vi "MathLink.vi"(2 "Arg":variant, 3 "Action":enum16{"Open", "Answer", "Close"}(ring), 4 "mlp in":u64) -> (0 "Status":i32, 1 "mlp out":u64)   [LabVIEW 2014]
uses:
  ml64i4.dll
panel:
  in  "VIs":variant
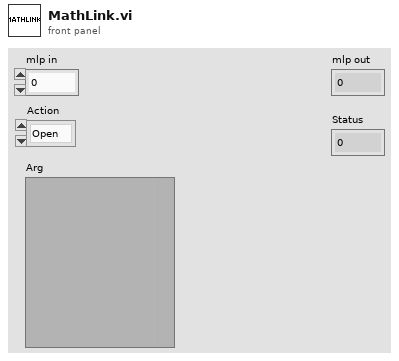
[diagram p1: front panel]
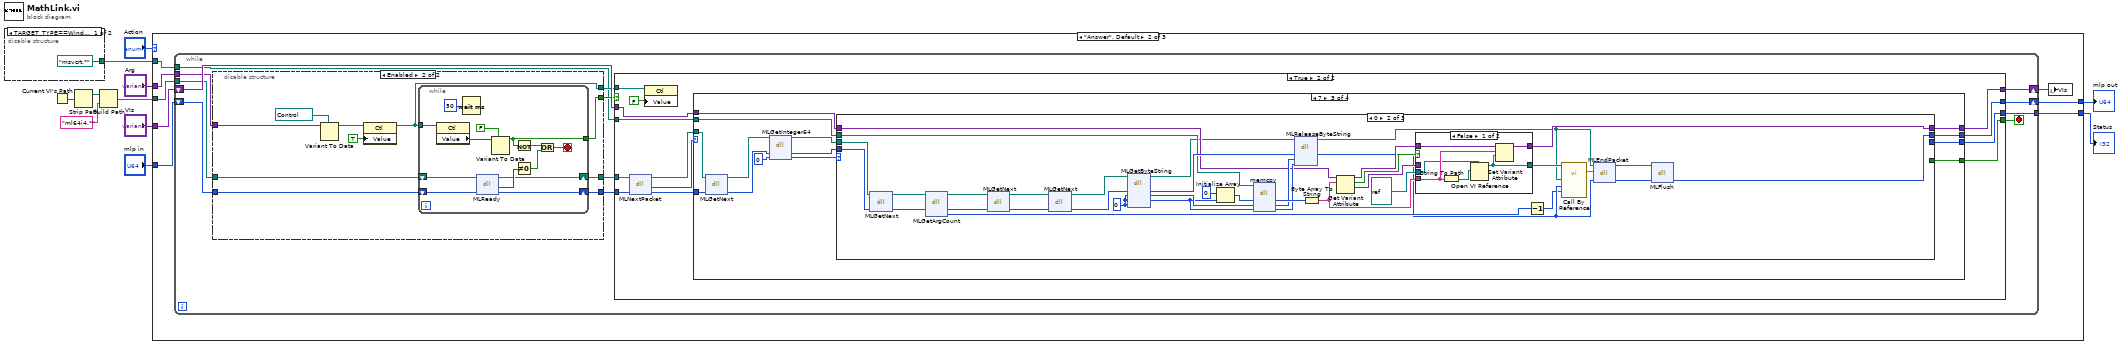
[diagram p0: block diagram]
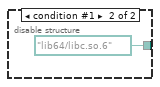
[diagram p2: hidden frame]
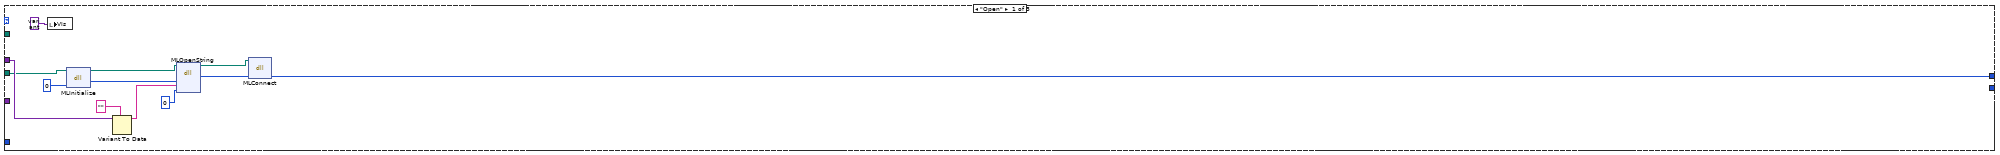
[diagram p3: hidden frame]
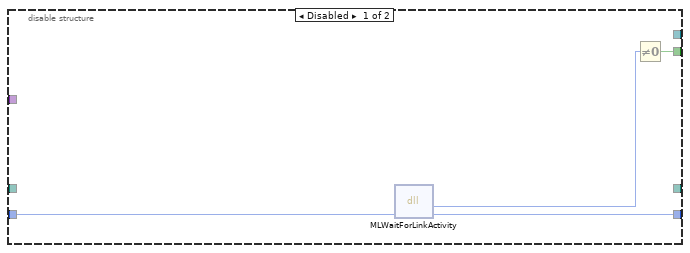
[diagram p4: hidden frame]
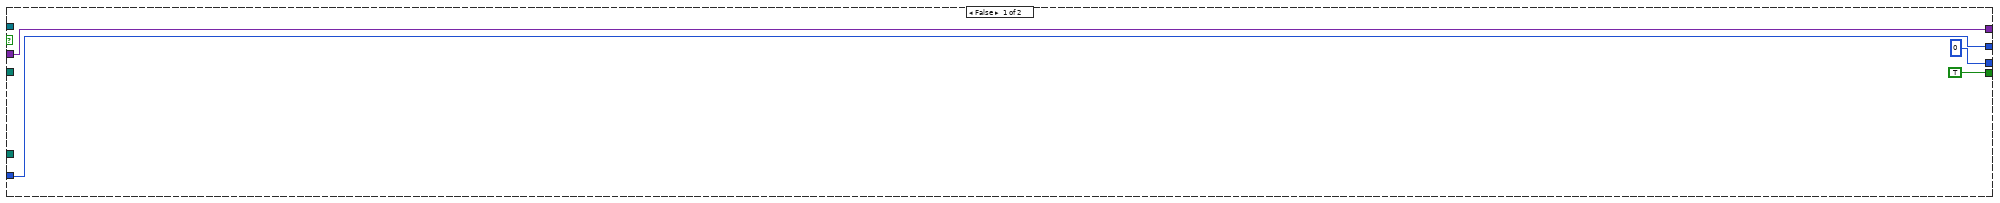
[diagram p5: hidden frame]
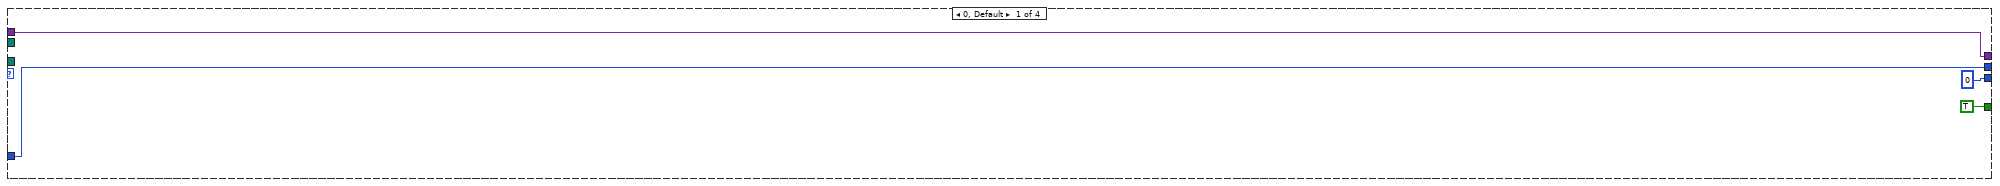
[diagram p6: hidden frame]
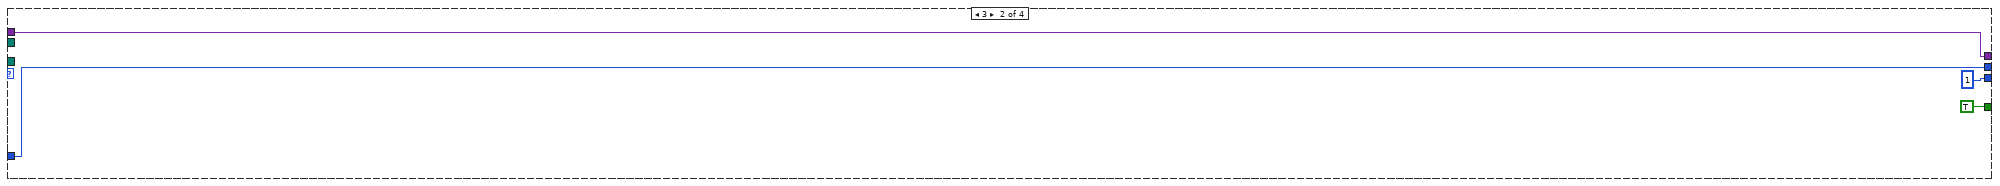
[diagram p7: hidden frame]
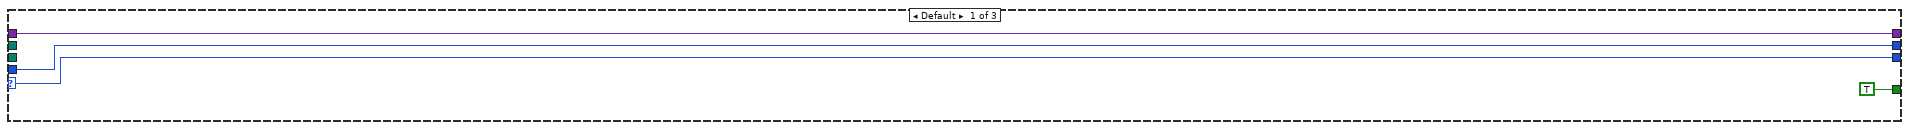
[diagram p8: hidden frame]
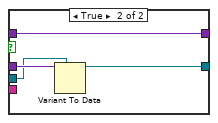
[diagram p9: hidden frame]
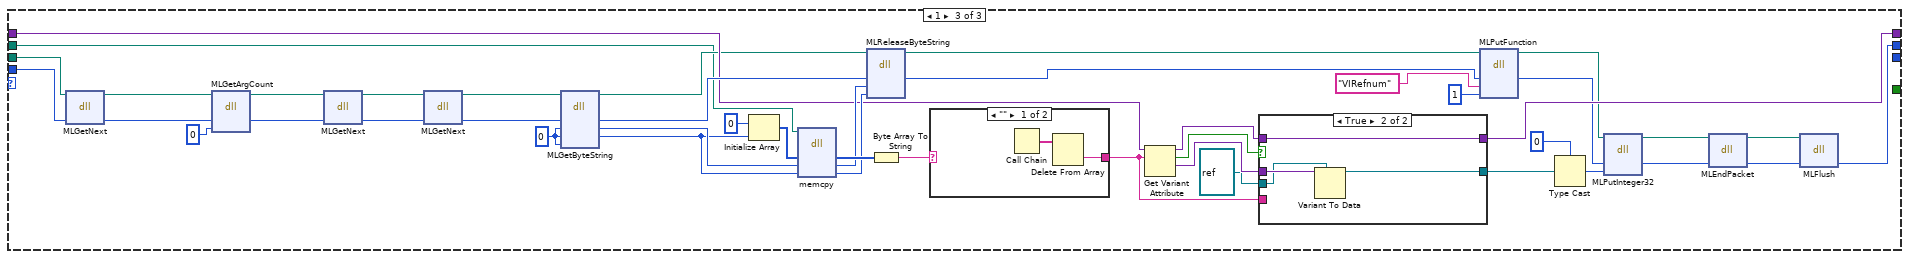
[diagram p10: hidden frame]
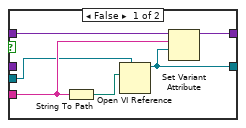
[diagram p12: hidden frame]
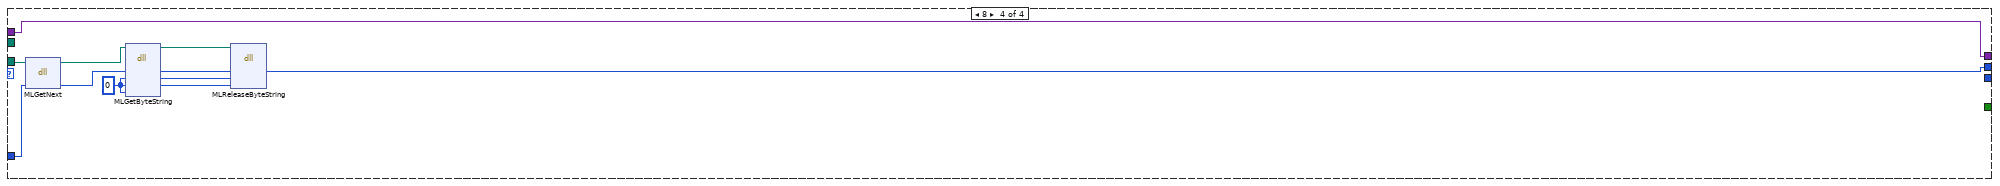
[diagram p13: hidden frame]
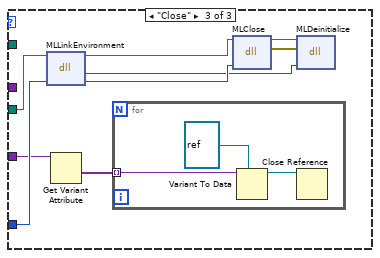
[diagram p14: hidden frame]
diagram:
  n1 = disable-structure shown="TARGET_TYPE==Windows, Default" {
    disable-tunnel: [path "msvcrt.*" ("path in") path "/lib64/libc.so.6" ("path in")] -> w1
    frame condition #0 (active) {
    }
    frame condition #1 {
    }
  }
  n2 = Current VI's Path() -> (path=w5:path)
  n3 = Strip Path(path=w5) -> (stripped path=w4:path)  [unwired: 1 out]
  n4 = Build Path(base path=w4, name or relative path="ml64i4.*") -> (appended path=w3:path)
  n5 = case shown="\"Answer\", Default" "Action" {
    tunnel: "Arg" -> [w19 w28 _]
    tunnel: [w21 w32 _] -> w10
    tunnel: "mlp in" -> [_ w33 w240]
    tunnel: [_ w31 _] -> w8
    tunnel: "VIs" -> [_ w29 w236]
    tunnel: w3 -> [w16 w27 w234]
    tunnel: w1 -> [_ w26 _]
    frame "Open" {
      n6 = local write "VIs"(variant ("VIs")) -> ()
      n7 = dll-call lib="ml64i4.dll" fn="MLInitialize"(path in=w16, "ep"=u64 0) -> (path out=w15:path, "env"=w24:u64)  [unwired: 3 in, 1 out]
      n8 = Variant To Data(type="" ("string"), Variant=w19) -> (data=w17:string)  [unwired: 1 in, 1 out]
      n9 = dll-call lib="ml64i4.dll" fn="MLOpenString"(path in=w15, "env"=w24, "cmd"=w17, "err"=0) -> (path out=w14:path, "mlp"=w22:u64)  [unwired: 5 in, 1 out]
      n10 = dll-call lib="ml64i4.dll" fn="MLConnect"(path in=w14, "mlp"=w22) -> ("mlp"=w21:u64)  [unwired: 3 in, 2 out]
    }
    frame "Answer", Default {
      n11 = while {
        shift-right: [w44] -> w32
        shift-left: w33 -> [w45]
        tunnel: [w42] -> w31
        shift-right: [w41] -> w30
        shift-left: w29 -> [w40]
        tunnel: w28 -> [w38]
        tunnel: w27 -> [w36]
        tunnel: w26 -> [w34]
        stop <- w43 stop-if-true
        n12 = disable-structure shown="Enabled" {
          disable-tunnel: [w50 w59] -> w46
          disable-tunnel: w45 -> [w49 w60]
          disable-tunnel: [w47 w58] -> w39
          disable-tunnel: w38 -> [_ w57]
          disable-tunnel: [_ w53] -> w37
          disable-tunnel: w36 -> [_ w52]
          disable-tunnel: [_ w51] -> w35
          frame Disabled {
            n13 = dll-call lib="ml64i4.dll" fn="MLWaitForLinkActivity"("mlp"=w49) -> (w48:i32, "mlp"=w50:u64)  [unwired: 3 in, 2 out]
            n14 = Not Equal To 0?(x=w48) -> (x != 0?=w47:bool)
          }
          frame Enabled {
            n15 = Variant To Data(type=refnum<vi> refnum ("Quit"), Variant=w57) -> (data=w55:refnum<vi>)  [unwired: 1 in, 1 out]
            n16 = property class="Ctl"(reference=w55, "Value"=TRUE ("x .or. y?")) -> (reference out=w53:refnum<vi>)  [unwired: 1 in, 1 out]
            n17 = while {
              shift-right: [w71] -> w59
              shift-left: w60 -> [w72]
              tunnel: w53 -> [w66]
              tunnel: [w63] -> w58
              shift-right: [w61] -> w51
              shift-left: w52 -> [w62]
              stop <- w68 stop-if-true
              n18 = property class="Ctl"(reference=w66) -> ("Value"=w65:variant)  [unwired: 1 in, 2 out]
              n19 = Wait (ms)(milliseconds to wait=u32 50) -> ()  [unwired: 1 out]
              n20 = dll-call lib="ml64i4.dll" fn="MLReady"(path in=w62, "mlp"=w72) -> (path out=w61:path, w73:i32, "mlp"=w71:u64)  [unwired: 2 in, 1 out]
              n21 = Variant To Data(type=FALSE ("x .or. y?"), Variant=w65) -> (data=w63:bool)  [unwired: 1 in, 1 out]
              n22 = Not(x=w63) -> (.not. x?=w67:bool)
              n23 = Not Equal To 0?(x=w73) -> (x != 0?=w69:bool)
              n24 = Or(x=w67, y=w69) -> (x .or. y?=w68:bool)
            }
          }
        }
        n25 = case shown="True" w39 {
          tunnel: w46 -> [w76 w90]
          tunnel: [w76 w87] -> w44
          tunnel: [TRUE w86] -> w43
          tunnel: [0 w85] -> w42
          tunnel: w40 -> [w74 w84]
          tunnel: [w74 w83] -> w41
          tunnel: w37 -> [_ w82]
          tunnel: w35 -> [_ w80]
          tunnel: w34 -> [_ w78]
          frame False {
          }
          frame True {
            n26 = dll-call lib="ml64i4.dll" fn="MLNextPacket"(path in=w80, "mlp"=w90) -> (path out=w79:path, w88:i32, "mlp"=w89:u64)  [unwired: 2 in, 1 out]
            n27 = property class="Ctl"(reference=w82, "Value"=FALSE ("x .or. y?")) -> ()  [unwired: 1 in, 2 out]
            n28 = case shown="7" w88 {
              tunnel: w89 -> [w92 w95 w110 w230]
              tunnel: [w92 w95 w106 w226] -> w87
              tunnel: [TRUE TRUE w109 _] -> w86
              tunnel: [i64 0 ("wp") 1 w108 _] -> w85
              tunnel: w84 -> [w91 w96 w105 w231]
              tunnel: [w91 w96 w104 w231] -> w83
              tunnel: w79 -> [_ _ w102 w223]
              tunnel: w78 -> [_ _ w99 _]
              frame 0, Default {
              }
              frame 3 {
              }
              frame 7 {
                n29 = dll-call lib="ml64i4.dll" fn="MLGetNext"(path in=w102, "mlp"=w110) -> (path out=w101:path, "mlp"=w111:u64)  [unwired: 3 in, 1 out]
                n30 = dll-call lib="ml64i4.dll" fn="MLGetInteger64"(path in=w101, "mlp"=w111, "wp"=i64 0) -> (path out=w100:path, "mlp"=w107:u64, "wp"=w103:i64)  [unwired: 3 in, 1 out]
                n31 = case shown="0" w103 {
                  selector: w103 -> [w115 _ _]
                  tunnel: [TRUE _ _] -> w109
                  tunnel: [w115 _ _] -> w108
                  tunnel: w107 -> [w114 w153 w207]
                  tunnel: [w114 w126 w175] -> w106
                  tunnel: w105 -> [w113 w135 w191]
                  tunnel: [w113 w134 w190] -> w104
                  tunnel: w100 -> [_ w125 w174]
                  tunnel: w99 -> [_ w120 w164]
                  frame Default {
                  }
                  frame 0 {
                    w144 = 0 ("len")
                    n32 = dll-call lib="ml64i4.dll" fn="MLGetNext"(path in=w125, "mlp"=w153) -> (path out=w124:path, "mlp"=w130:u64)  [unwired: 3 in, 1 out]
                    n33 = dll-call lib="ml64i4.dll" fn="MLGetArgCount"(path in=w124, "mlp"=w130) -> (path out=w123:path, "mlp"=w152:u64, "countp"=w131:i32)  [unwired: 4 in, 1 out]
                    n34 = dll-call lib="ml64i4.dll" fn="MLGetNext"(path in=w123, "mlp"=w152) -> (path out=w122:path, "mlp"=w138:u64)  [unwired: 3 in, 1 out]
                    n35 = dll-call lib="ml64i4.dll" fn="MLGetNext"(path in=w122, "mlp"=w138) -> (path out=w121:path, "mlp"=w137:u64)  [unwired: 3 in, 1 out]
                    n36 = dll-call lib="ml64i4.dll" fn="MLGetByteString"(path in=w121, "mlp"=w137, "bufp"=w144, "lenp"=w144, "missing"=w144) -> (path out=w119:path, "mlp"=w141:u64, "bufp"=w143:u64, "lenp"=w142:i32)  [unwired: 4 in, 1 out]
                    n37 = Initialize Array(u8 0 ("element"), w142) -> (w146:u8[])
                    n38 = dll-call lib="lib64/libc.so.6" fn="memcpy"(path in=w120, "dest"=w146, "src"=w143, "size"=w142) -> ("dest"=w145:u8[], "src"=w140:u64, "size"=w139:i32)  [unwired: 3 in, 2 out]
                    n39 = dll-call lib="ml64i4.dll" fn="MLReleaseByteString"(path in=w119, "mlp"=w141, "buf"=w140, "len"=w139) -> (path out=w117:path, "mlp"=w129:u64)  [unwired: 5 in, 1 out]
                    n40 = Byte Array To String(unsigned byte array=w145) -> (string=w136:string)
                    n41 = Get Variant Attribute(Variant=w135, name=w136) -> (duplicate Variant=w149:variant, found=w151:bool, value=w150:variant)  [unwired: 2 in, 1 out]
                    n42 = case shown="False" w151 {
                      tunnel: w136 -> [w159 _]
                      tunnel: w150 -> [_ w163]
                      tunnel: w149 -> [w156 w162]
                      tunnel: [w154 w160] -> w133
                      tunnel: refnum<vi> refnum ("type specifier VI Refnum (for type only)") -> [w157 w161]
                      tunnel: [w155 w162] -> w134
                      frame False {
                        n43 = String To Path(string=w159) -> (path=w158:path)
                        n44 = Open VI Reference(type specifier VI Refnum (for type only)=w157, vi path=w158) -> (vi reference=w154:refnum<vi>)  [unwired: 4 in, 1 out]
                        n45 = Set Variant Attribute(Variant=w156, name=w159, value=w154) -> (Variant out=w155:variant)  [unwired: 1 in, 2 out]
                      }
                      frame True {
                        n46 = Variant To Data(type=w161, Variant=w163) -> (data=w160:refnum<vi>)  [unwired: 1 in, 1 out]
                      }
                    }
                    n47 = Decrement(x=w131) -> (x-1=w128:i32)
                    n48 = call-by-ref "?"(reference=w133, "n"=w128, "mlp"=w129, "MathLink Dll"=w117) -> (error out=w132:errorcluster)  [unwired: 1 in, 1 out]
                    n49 = dll-call lib="ml64i4.dll" fn="MLEndPacket"(path in=w117, error in=w132, "mlp"=w129) -> (path out=w118:path, "mlp"=w127:u64)  [unwired: 2 in, 1 out]
                    n50 = dll-call lib="ml64i4.dll" fn="MLFlush"(path in=w118, "mlp"=w127) -> ("mlp"=w126:u64)  [unwired: 3 in, 2 out]
                  }
                  frame 1 {
                    w199 = 0 ("len")
                    n51 = dll-call lib="ml64i4.dll" fn="MLGetNext"(path in=w174, "mlp"=w207) -> (path out=w173:path, "mlp"=w178:u64)  [unwired: 3 in, 1 out]
                    n52 = dll-call lib="ml64i4.dll" fn="MLGetArgCount"(path in=w173, "mlp"=w178, "countp"=0) -> (path out=w172:path, "mlp"=w206:u64)  [unwired: 4 in, 1 out]
                    n53 = dll-call lib="ml64i4.dll" fn="MLGetNext"(path in=w172, "mlp"=w206) -> (path out=w171:path, "mlp"=w193:u64)  [unwired: 3 in, 1 out]
                    n54 = dll-call lib="ml64i4.dll" fn="MLGetNext"(path in=w171, "mlp"=w193) -> (path out=w170:path, "mlp"=w192:u64)  [unwired: 3 in, 1 out]
                    n55 = dll-call lib="ml64i4.dll" fn="MLGetByteString"(path in=w170, "mlp"=w192, "bufp"=w199, "lenp"=w199, "missing"=w199) -> (path out=w169:path, "mlp"=w196:u64, "bufp"=w198:u64, "lenp"=w197:i32)  [unwired: 4 in, 1 out]
                    n56 = Initialize Array(u8 0 ("element"), w197) -> (w201:u8[])
                    n57 = dll-call lib="lib64/libc.so.6" fn="memcpy"(path in=w164, "dest"=w201, "src"=w198, "size"=w197) -> ("dest"=w200:u8[], "src"=w195:u64, "size"=w194:i32)  [unwired: 3 in, 2 out]
                    n58 = dll-call lib="ml64i4.dll" fn="MLReleaseByteString"(path in=w169, "mlp"=w196, "buf"=w195, "len"=w194) -> (path out=w168:path, "mlp"=w187:u64)  [unwired: 5 in, 1 out]
                    n59 = Byte Array To String(unsigned byte array=w200) -> (string=w180:string)
                    n60 = case shown="\"\"" w180 {
                      selector: w180 -> [_ w210]
                      tunnel: [w208 w210] -> w179
                      frame "" {
                        n61 = Call Chain() -> (call chain=w209:string[])
                        n62 = Delete From Array(array=w209) -> (deleted portion=w208:string)  [unwired: 2 in, 1 out]
                      }
                      frame Default {
                      }
                    }
                    n63 = Get Variant Attribute(Variant=w191, name=w179) -> (duplicate Variant=w203:variant, found=w205:bool, value=w204:variant)  [unwired: 2 in, 1 out]
                    n64 = case shown="True" w205 {
                      tunnel: w179 -> [w216 _]
                      tunnel: w204 -> [_ w220]
                      tunnel: w203 -> [w213 w219]
                      tunnel: [w211 w217] -> w182
                      tunnel: refnum<vi> refnum ("vi reference") -> [w214 w218]
                      tunnel: [w212 w219] -> w190
                      frame False {
                        n65 = String To Path(string=w216) -> (path=w215:path)
                        n66 = Open VI Reference(type specifier VI Refnum (for type only)=w214, vi path=w215) -> (vi reference=w211:refnum<vi>)  [unwired: 4 in, 1 out]
                        n67 = Set Variant Attribute(Variant=w213, name=w216, value=w211) -> (Variant out=w212:variant)  [unwired: 1 in, 2 out]
                      }
                      frame True {
                        n68 = Variant To Data(type=w218, Variant=w220) -> (data=w217:refnum<vi>)  [unwired: 1 in, 1 out]
                      }
                    }
                    n69 = dll-call lib="ml64i4.dll" fn="MLPutFunction"(path in=w168, "mlp"=w187, "s"="VIRefnum", "argc"=1) -> (path out=w167:path, "mlp"=w189:u64)  [unwired: 5 in, 1 out]
                    n70 = Type Cast(type=u32 0 ("i"), x=w182) -> (*(type *) &x=w181:u32)
                    n71 = dll-call lib="ml64i4.dll" fn="MLPutInteger32"(path in=w167, "mlp"=w189, "i"=w181) -> (path out=w166:path, "mlp"=w186:u64)  [unwired: 4 in, 1 out]
                    n72 = dll-call lib="ml64i4.dll" fn="MLEndPacket"(path in=w166, "mlp"=w186) -> (path out=w165:path, "mlp"=w176:u64)  [unwired: 3 in, 1 out]
                    n73 = dll-call lib="ml64i4.dll" fn="MLFlush"(path in=w165, "mlp"=w176) -> ("mlp"=w175:u64)  [unwired: 3 in, 2 out]
                  }
                }
              }
              frame 8 {
                w229 = 0 ("len")
                n74 = dll-call lib="ml64i4.dll" fn="MLGetNext"(path in=w223, "mlp"=w230) -> (path out=w222:path, "mlp"=w227:u64)  [unwired: 3 in, 1 out]
                n75 = dll-call lib="ml64i4.dll" fn="MLGetByteString"(path in=w222, "mlp"=w227, "bufp"=w229, "lenp"=w229, "missing"=w229) -> (path out=w221:path, "mlp"=w228:u64, "bufp"=w225:u64, "lenp"=w224:i32)  [unwired: 4 in, 1 out]
                n76 = dll-call lib="ml64i4.dll" fn="MLReleaseByteString"(path in=w221, "mlp"=w228, "buf"=w225, "len"=w224) -> ("mlp"=w226:u64)  [unwired: 5 in, 2 out]
              }
            }
          }
        }
      }
      n77 = local write "VIs"(w30) -> ()
    }
    frame "Close" {
      n78 = dll-call lib="ml64i4.dll" fn="MLLinkEnvironment"(path in=w234, "mlp"=w240) -> (path out=w233:path, "env"=w238:u64, "mlp"=w239:u64)  [unwired: 2 in, 1 out]
      n79 = Get Variant Attribute(Variant=w236) -> (values=w235:variant[])  [unwired: 3 in, 3 out]
      n80 = for {
        tunnel: w235 -> [w242] mode=indexing
        n81 = Variant To Data(type=refnum<vi> refnum ("vi reference"), Variant=w242) -> (data=w241:refnum<vi>)  [unwired: 1 in, 1 out]
        n82 = Close Reference(reference=w241) -> ()  [unwired: 1 in, 1 out]
      }
      n83 = dll-call lib="ml64i4.dll" fn="MLClose"(path in=w233, "mlp"=w239) -> (path out=w232:path, error out=w237:errorcluster)  [unwired: 4 in]
      n84 = dll-call lib="ml64i4.dll" fn="MLDeinitialize"(path in=w232, error in=w237, "env"=w238) -> ()  [unwired: 3 in, 2 out]
    }
  }
  "mlp out" <- w10
  "Status" <- w8
